vi "Report Type.vi"(0 "report in":refnum<class "NI_Excel.lvclass">, 11 "error in (no error)":errorcluster) -> (4 "report out":refnum<class "NI_Excel.lvclass">, 8 "report type":T1, 15 "error out":errorcluster)   [LabVIEW 2020, in "NI_Excel.lvclass"]
doc: "Returns the report type, such as standard on Windows, or HTML on all platforms, of a specified report.\n\nThis VI also returns Microsoft Word or Excel report types."
uses:
  <vilib>/Utility/NIReport.llb/Excel/NI_Excel.lvclass
  <vilib>/Utility/NIReport.llb/Report Type.ctl
  <vilib>/Utility/NIReport.llb/NI_ReportGenerationCore.lvlib
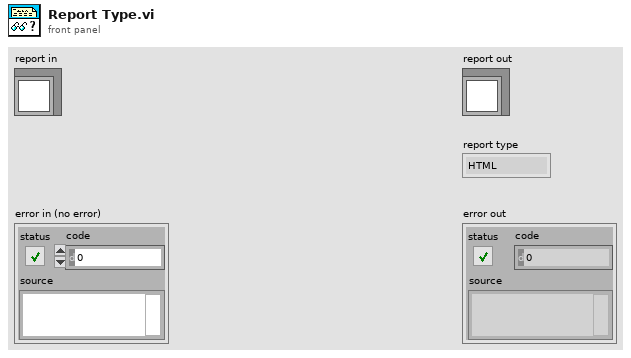
[diagram p1: front panel]
types:
  T1 = typedef "NI_ReportGenerationCore.lvlib/Report Type.ctl" = enum16{"HTML", "Word", "Excel"}
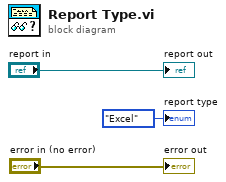
[diagram p0: block diagram]
diagram:
  "error out" <- "error in (no error)"
  "report out" <- "report in"
  "report type" <- Report_Type."Excel" ("report type")
